vi "Configure Arbitrary Waveform [ARB] Core.vi"(5 "offset (0.00 V)":dbl[unit] format="%.4f", 7 "gain (1.00)":dbl=1.0 format="%.4f", 8 "error in (no error)":errorcluster, 9 "waveform handle (0)":i32, 10 "channel name (\"CHANNEL1\")":string="CHANNEL1", 11 "IVI_Fgen in":refnum<class "IVI_Fgen.lvclass">) -> (0 "error out":errorcluster, 3 "IVI_Fgen out":refnum<class "IVI_Fgen.lvclass">)   [LabVIEW 2013, in "IVI_Fgen.lvlib" / "IVI_Fgen.lvclass"]
doc: "This VI configures the properties of the function generator that affect arbitrary waveform generation. These properties are the arbitrary waveform handle, gain, and offset.\n\nNotes:\n\n(1) This VI is part of the IviFgenArbWfm [ARB] extension group."
uses:
  IVI_Fgen.lvclass
  IVI_Fgen.lvclass/IVI_Fgen.ctl
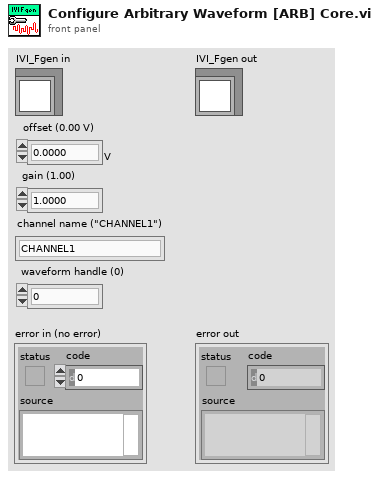
[diagram p1: front panel]
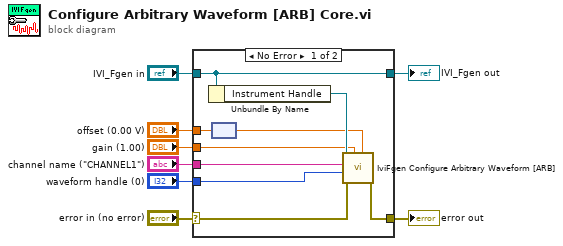
[diagram p0: block diagram]
diagram:
  n1 = case shown="No Error" "error in (no error)" {
    selector: "error in (no error)" -> [w15 w19]
    tunnel: [w14 w19] -> w7
    tunnel: [w17 w18] -> w5
    tunnel: "IVI_Fgen in" -> [w17 w18]
    tunnel: "channel name (\"CHANNEL1\")" -> [w13 _]
    tunnel: "offset (0.00 V)" -> [w12 _]
    tunnel: "gain (1.00)" -> [w9 _]
    tunnel: "waveform handle (0)" -> [w11 _]
    frame No Error {
      n2 = Unbundle By Name(w17) -> ("Instrument Handle"=w16:refnum<k15>)
      n3 = node(w12) -> (w10:dbl)
      n4 = call <vilib>:"IviFgen Configure Arbitrary Waveform [ARB].vi"("offset (0.00 V)"=w10, "gain (1.00)"=w9, "error in (no error)"=w15, "waveform handle (0)"=w11, "channel name (\"CHANNEL1\")"=w13, "instrument handle"=w16) -> ("error out"=w14:errorcluster)  [unwired: 4 in, 1 out]
    }
    frame Error {
    }
  }
  "error out" <- w7
  "IVI_Fgen out" <- w5
